vi "Generate Joint Trajectory (Array).vi"(4 "end joint velocities":dbl[](array[numeric]), 6 "start joint velocities":dbl[](array[numeric]), 7 "intermediate points":dbl[](array[numeric]), 8 "error in (no error)":errorcluster, 10 "end joint positions":dbl[](array[numeric]), 11 "start joint positions":dbl[](array[numeric])) -> (0 "error out":errorcluster, 1 "joint acceleration trajectory":dbl[][](array[numeric]), 2 "joint velocity trajectory":dbl[][](array[numeric]), 3 "joint position trajectory":dbl[][](array[numeric]))   [LabVIEW 2017, in "NI_Kinematics.lvlib"]
doc: "Generates joint angles, velocities, and accelerations along a smooth trajectory between two points in joint space. Wire data to the <B>intermediate points</B> input to determine the polymorphic instance to use or manually select the instance.\n\n<B>.m file:</B> jtraj"
uses:
  <vilib>/robotics/Kinematics/NI_Kinematics.lvlib
  <vilib>/Analysis/Matrix/Datatypes/RealMatrix.ctl
  <vilib>/Analysis/baseanly.llb/Real A x B.vi
  <vilib>/Analysis/NI_AALBase.lvlib
  <vilib>/Analysis/Matrix/NI_Matrix.lvlib
  <vilib>/robotics/Utilities/NI_Robotics Utilities.lvlib
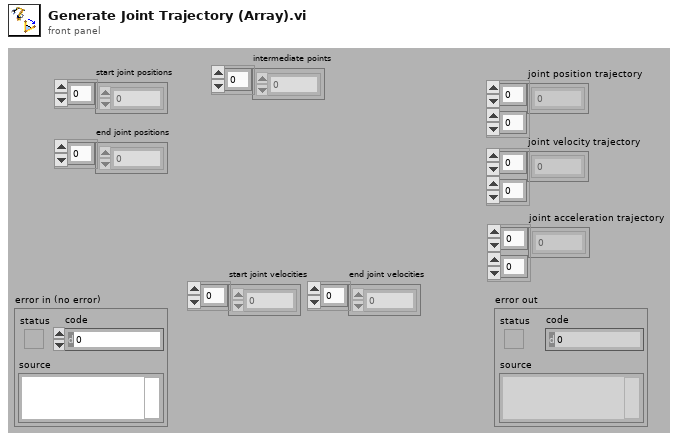
[diagram p1: front panel]
types:
  T1 = typedef "NI_Matrix.lvlib/RealMatrix.ctl" = dbl[][]
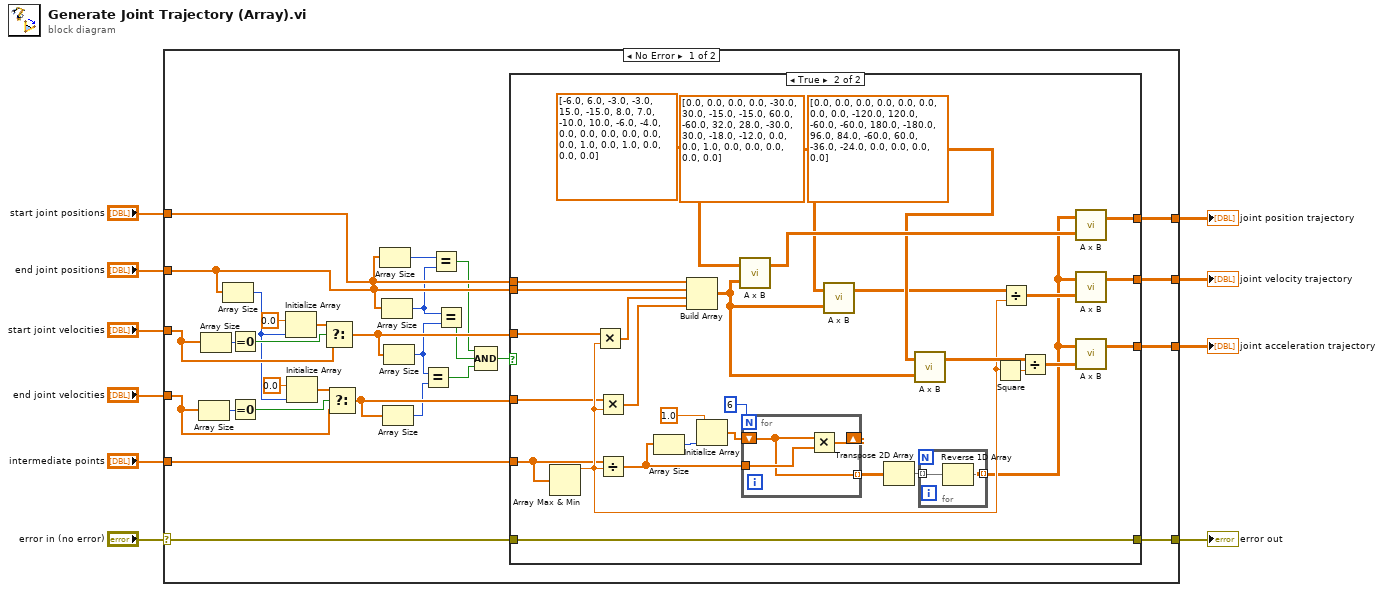
[diagram p0: block diagram]
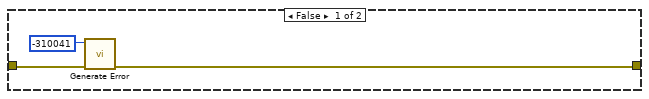
[diagram p2: hidden frame]
diagram:
  n1 = case shown="No Error" "error in (no error)" {
    selector: "error in (no error)" -> [w12 w78]
    tunnel: [w39 _] -> w10
    tunnel: [w38 _] -> w9
    tunnel: [w37 _] -> w8
    tunnel: "end joint velocities" -> [w28 _]
    tunnel: "start joint velocities" -> [w27 _]
    tunnel: "end joint positions" -> [w23 _]
    tunnel: "start joint positions" -> [w22 _]
    tunnel: [w14 w78] -> w3
    tunnel: "intermediate points" -> [w11 _]
    frame No Error {
      n2 = Array Size(array=w28) -> (size(s)=w30:i32)
      n3 = Array Size(array=w27) -> (size(s)=w36:i32)
      n4 = Array Size(array=w23) -> (size(s)=w26:i32)
      n5 = Equal To 0?(x=w36) -> (x = 0?=w35:bool)
      n6 = Equal To 0?(x=w30) -> (x = 0?=w29:bool)
      n7 = Initialize Array(0.0, w26) -> (w34:dbl[])
      n8 = Initialize Array(0.0, w26) -> (w31:dbl[])
      n9 = Select(t=w34, s=w35, f=w27) -> (s? t:f=w25:dbl[])
      n10 = Select(t=w31, s=w29, f=w28) -> (s? t:f=w24:dbl[])
      n11 = Array Size(array=w22) -> (size(s)=w21:i32)
      n12 = Array Size(array=w23) -> (size(s)=w19:i32)
      n13 = Array Size(array=w24) -> (size(s)=w20:i32)
      n14 = Array Size(array=w25) -> (size(s)=w18:i32)
      n15 = Equal?(x=w18, y=w20) -> (x = y?=w15:bool)
      n16 = Equal?(x=w21, y=w19) -> (x = y?=w17:bool)
      n17 = Equal?(x=w19, y=w18) -> (x = y?=w16:bool)
      n18 = Compound Arithmetic op=AND(w17, w16, w15) -> (w13:bool)
      n19 = case shown="True" w13 {
        tunnel: [_ w63] -> w39
        tunnel: [_ w61] -> w38
        tunnel: [_ w60] -> w37
        tunnel: w25 -> [_ w48]
        tunnel: w24 -> [_ w47]
        tunnel: w23 -> [_ w46]
        tunnel: w22 -> [_ w45]
        tunnel: w12 -> [w41 w44]
        tunnel: [w40 w44] -> w14
        tunnel: w11 -> [_ w43]
        frame False {
          n20 = call <vilib>:"Generate Error.vi"("error in (no error)"=w41, "code"=-310041) -> ("error out"=w40:errorcluster)  [unwired: 9 in]
        }
        frame True {
          n21 = Array Max & Min(array=w43) -> (max value=w53:dbl)  [unwired: 3 out]
          n22 = Multiply(x=w48, y=w53) -> (x*y=w71:dbl[])
          n23 = Multiply(x=w47, y=w53) -> (x*y=w72:dbl[])
          n24 = Divide(x=w43, y=w53) -> (x/y=w68:dbl[])
          n25 = Array Size(array=w68) -> (size(s)=w67:i32)
          n26 = Build Array(w45, w46, w71, w72) -> (w59:T1)
          n27 = Initialize Array(1.0 ("element"), w67) -> (w65:dbl[])
          n28 = call-poly <vilib>:"A x B.vi"("B"=w59, "A"=T1 [[-6.0, 6.0, -3.0, -3.0], [15.0, -15.0, 8.0, 7.0], [-10.0, 10.0, -6.0, -4.0], [0.0, 0.0, 0.0, 0.0], [0.0, 0.0, 1.0, 0.0], [1.0, 0.0, 0.0, 0.0]]) -> ("A x B"=w64:T1)  [unwired: 1 out]
          n29 = for {
            N: 6 -> [_]
            shift-right: [w75] -> _
            shift-left: w65 -> [w76]
            tunnel: w68 -> [w77]
            tunnel: [w76] -> w51 mode=indexing
            n30 = Multiply(x=w76, y=w77) -> (x*y=w75:dbl[])
          }
          n31 = call-poly <vilib>:"A x B.vi"("B"=w59, "A"=T1 [[0.0, 0.0, 0.0, 0.0], [-30.0, 30.0, -15.0, -15.0], [60.0, -60.0, 32.0, 28.0], [-30.0, 30.0, -18.0, -12.0], [0.0, 0.0, 1.0, 0.0], [0.0, 0.0, 0.0, 0.0]]) -> ("A x B"=w52:T1)  [unwired: 1 out]
          n32 = Transpose 2D Array(2D array=w51) -> (transposed array=w50:dbl[][])
          n33 = call-poly <vilib>:"A x B.vi"("B"=w59, "A"=T1 [[0.0, 0.0, 0.0, 0.0], [0.0, 0.0, 0.0, 0.0], [-120.0, 120.0, -60.0, -60.0], [180.0, -180.0, 96.0, 84.0], [-60.0, 60.0, -36.0, -24.0], [0.0, 0.0, 0.0, 0.0]]) -> ("A x B"=w57:T1)  [unwired: 1 out]
          n34 = for {
            tunnel: [w74] -> w49 mode=indexing
            tunnel: w50 -> [w73] mode=indexing
            n35 = Reverse 1D Array(array=w73) -> (reversed array=w74:dbl[])
          }
          n36 = Square(x=w53) -> (x^2=w54:dbl)
          n37 = Divide(x=w52, y=w53) -> (x/y=w55:T1)
          n38 = Divide(x=w57, y=w54) -> (x/y=w56:T1)
          n39 = call-poly <vilib>:"A x B.vi"("B"=w64, "A"=w49) -> ("A x B"=w63:T1)  [unwired: 1 out]
          n40 = call-poly <vilib>:"A x B.vi"("B"=w55, "A"=w49) -> ("A x B"=w61:T1)  [unwired: 1 out]
          n41 = call-poly <vilib>:"A x B.vi"("B"=w56, "A"=w49) -> ("A x B"=w60:T1)  [unwired: 1 out]
        }
      }
    }
    frame Error {
    }
  }
  "joint position trajectory" <- w10
  "joint velocity trajectory" <- w9
  "joint acceleration trajectory" <- w8
  "error out" <- w3
